vi "Data.vi"(11 "Destroy Msg in":refnum<class "Destroy Msg.lvclass">) -> ()   [LabVIEW 2021, in "Destroy.lvlib" / "Destroy Msg.lvclass"]
uses:
  Destroy Msg.lvclass
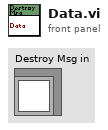
[diagram p1: front panel]
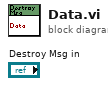
[diagram p0: block diagram]
diagram:
